vi "I(V)_MFLI_PK_v4.0_measureR_phase.vi"() -> ()   [LabVIEW 2016]
uses:
  Labview Drivers/MFLI/LabOneLabVIEW-22.02.26577/LabOneLabVIEW-22.02.26577/Zurich Instruments LabOne/Public/Data/ziTypeDemodSampleSingle.ctl
  Labview Drivers/MFLI/LabOneLabVIEW-22.02.26577/LabOneLabVIEW-22.02.26577/Zurich Instruments LabOne/Public/Configure/ziSetValueDouble.vi
  Labview Drivers/MFLI/LabOneLabVIEW-22.02.26577/LabOneLabVIEW-22.02.26577/Zurich Instruments LabOne/Public/Configure/ziGetValueDemodSampleEx.vi
  Labview Drivers/MFLI/LabOneLabVIEW-22.02.26577/LabOneLabVIEW-22.02.26577/Zurich Instruments LabOne/Zurich Instruments LabOne.lvlib
panel:
  out "Iphase (deg)":dbl=-16.59997463839791 format="%#_13g"
  out "Vphase (deg)":dbl=40.57455732074348 format="%#_13g"
  out "Set Voltage(V)":dbl=4.384062043356605 format="%#_13g"
  out "Time(s)":dbl=185.322 format="%#_13g"
  out "Demod Sample Out 2":T1={"Timestamps (ticks)"=217071890701310, "X (Vrms)"=5.764492493379272e-06, "Y (Vrms)"=-1.7187028687058897e-06, "Osc Phase (deg)"=1.9746167692057917, "Freq (Hz)"=7.919000069023241, "DIO"=0, "AuxIn0 (V)"=-0.0006693530012853444, "AuxIn1 (V)"=0.0, "Trigger"=256}
  out "Demod Sample Out":T1={"Timestamps (ticks)"=217071887690750, "X (Vrms)"=8.75456933556226e-07, "Y (Vrms)"=7.498226005787958e-07, "Osc Phase (deg)"=5.4774618983426535, "Freq (Hz)"=7.919000069023241, "DIO"=0, "AuxIn0 (V)"=-0.001673382503213361, "AuxIn1 (V)"=-0.0006673162570223212, "Trigger"=512}
  in  "MFLI Current source/Voltage reader":string="DEV4496"
  out "Imeas (A)":dbl=6.015256707500007e-06
  out "Vmeas (V)":dbl=1.1526746179431637e-06
  in  "Folder":path=path "D:/Heng/Nb3Br8_JJ/Sb.3_NBVJ01/20210115"
  in  "wait (ms) [Should be > TC]":u32=1000
  out "I vs V":cluster{dbl, "Field Reading":dbl}[](graph)=[{2.1337108522522826e-07, "Field Reading"=1.0007121497539348e-06}, {2.0018204953851064e-08, "Field Reading"=1.0969598663661376e-07}, {3.474074033482476e-08, "Field Reading"=1.9016075130631681e-07}, {5.6400419155691035e-08, "Field Reading"=2.706780203266455e-07}, {7.134741663483111e-08, "Field Reading"=3.625194153695155e-07}, {8.711957733763268e-08, "Field Reading"=4.6186456260881066e-07}, {1.039613386460647e-07, "Field Reading"=5.541771498802743e-07}, {1.290159481540569e-07, "Field Reading"=6.517488283090827e-07}, {1.442006622421336e-07, "Field Reading"=7.441421685111633e-07}, {1.6579779771841864e-07, "Field Reading"=8.4200282004452e-07}, {1.7667431320194624e-07, "Field Reading"=9.371894272094692e-07}, {2.0346799660082097e-07, "Field Reading"=1.0346819690568719e-06}, {2.1275449478314156e-07, "Field Reading"=1.1273455634288892e-06}, {2.2792303722372882e-07, "Field Reading"=1.2246113813938451e-06}, {2.506226161778463e-07, "Field Reading"=1.3169699353558023e-06}, {2.6686786096204173e-07, "Field Reading"=1.4106741902497636e-06}, {2.979630377408132e-07, "Field Reading"=1.5068897992871093e-06}, {3.1162936250255217e-07, "Field Reading"=1.6013785409354697e-06}, {3.2854904168138843e-07, "Field Reading"=1.7007967107121696e-06}, {3.4501678279448686e-07, "Field Reading"=1.7932741209540488e-06}, {3.5732655253185603e-07, "Field Reading"=1.891133061059139e-06}, {3.7678513716337806e-07, "Field Reading"=1.9837632139333797e-06}, {3.8857693765173823e-07, "Field Reading"=2.078638757139878e-06}, {4.070455630330932e-07, "Field Reading"=2.1777621608691614e-06}, {4.3651006057087547e-07, "Field Reading"=2.270487653250022e-06}, {4.535609885287045e-07, "Field Reading"=2.364817703267964e-06}, {4.800092323465329e-07, "Field Reading"=2.4630513126122318e-06}, {4.872172260420143e-07, "Field Reading"=2.560612214294704e-06}, {5.029105394973937e-07, "Field Reading"=2.653407522930296e-06}, {5.207137968885614e-07, "Field Reading"=2.7508846993110185e-06}, {5.449974912672081e-07, "Field Reading"=2.8437164663468094e-06}, {5.549097834910874e-07, "Field Reading"=2.941117576580943e-06}, {5.789147944756835e-07, "Field Reading"=3.0334756142859178e-06}, {5.940331669154695e-07, "Field Reading"=3.130923358288321e-06}, {6.192662248173834e-07, "Field Reading"=3.223457045619671e-06}, {6.338859460756282e-07, "Field Reading"=3.3210140787077685e-06}, {6.617730672082958e-07, "Field Reading"=3.4134337904467758e-06}, {6.708744764433933e-07, "Field Reading"=3.511218639909905e-06}, {6.876034184888421e-07, "Field Reading"=3.6064791588715936e-06}, {7.081705825683568e-07, "Field Reading"=3.704194984998823e-06}, {7.341349902267621e-07, "Field Reading"=3.796795088130521e-06}, {7.500412173627324e-07, "Field Reading"=3.894221622472711e-06}, {7.635282212201655e-07, "Field Reading"=3.986359362120525e-06}, {7.839559208505005e-07, "Field Reading"=4.084105589459172e-06}, {7.991337007295971e-07, "Field Reading"=4.176440151889332e-06}, {8.175550663233945e-07, "Field Reading"=4.274041338897146e-06}, {8.360511976155764e-07, "Field Reading"=4.366718612721536e-06}, {8.595654269642977e-07, "Field Reading"=4.46481586459238e-06}, {8.846044621269243e-07, "Field Reading"=4.559710869350914e-06}, {8.902214589762566e-07, "Field Reading"=4.6535858762473605e-06}, {9.13930972707384e-07, "Field Reading"=4.751211544539011e-06}, {9.218629476317926e-07, "Field Reading"=4.843674806906942e-06}, {9.389346568153207e-07, "Field Reading"=4.94148963023105e-06}, {9.661788530141893e-07, "Field Reading"=5.0340339305698605e-06}, {9.734275114489362e-07, "Field Reading"=5.134274890899915e-06}, {9.91273930192609e-07, "Field Reading"=5.227194198108034e-06}, {1.0062090937222443e-06, "Field Reading"=5.324543514118811e-06}, {1.0324830232331714e-06, "Field Reading"=5.417068558459935e-06}, {1.0500453704719826e-06, "Field Reading"=5.514414049876445e-06}, {1.0818020141498576e-06, "Field Reading"=5.606738838727315e-06}, {1.0919981214621985e-06, "Field Reading"=5.943499955969014e-06}, {1.1041062115858416e-06, "Field Reading"=5.802825671371831e-06}, {1.12928896400331e-06, "Field Reading"=5.8897635364887065e-06}, {1.1492595887607054e-06, "Field Reading"=5.986959246668246e-06}, {1.1525838773614565e-06, "Field Reading"=6.079112281920131e-06}, {1.1732006667255544e-06, "Field Reading"=6.176765549637453e-06}, {1.193444625294635e-06, "Field Reading"=6.2693583656248445e-06}, {1.2101538188023656e-06, "Field Reading"=6.369277338631168e-06}, {1.2318147585414787e-06, "Field Reading"=6.462177680852612e-06}, {1.2413491771177379e-06, "Field Reading"=6.554239754143973e-06}, {1.2731631837142253e-06, "Field Reading"=6.653541226069562e-06}, {1.2825564782833625e-06, "Field Reading"=6.7454110623267924e-06}, {1.2992348301055137e-06, "Field Reading"=6.843115368447837e-06}, {1.316693256967963e-06, "Field Reading"=6.935702965257668e-06}, {1.343852132299077e-06, "Field Reading"=7.033596304342718e-06}, {0.0003223256295561193, "Field Reading"=7.130369502789653e-06}, {0.0010682796466779994, "Field Reading"=7.237712618778445e-06}, {0.0011012721847992696, "Field Reading"=7.315133567183911e-06}, {0.0011336841810168491, "Field Reading"=7.4123545054478695e-06}, {0.0011614058556892847, "Field Reading"=7.504304430827025e-06}, {0.001182885890671154, "Field Reading"=7.602366955750201e-06}, {0.001200897535521615, "Field Reading"=7.69976061587441e-06}, {0.00121594401470624, "Field Reading"=7.792677109208386e-06}, {0.0012308027651267619, "Field Reading"=7.886128685028496e-06}, {0.0012456418637471253, "Field Reading"=7.983615236672288e-06}, {0.001257564969772003, "Field Reading"=8.075760842161778e-06}, {0.0012690336996615858, "Field Reading"=8.170723157183957e-06}, {0.0012814644345765262, "Field Reading"=8.268995175290895e-06}, {0.0012910253378675095, "Field Reading"=8.363131378141633e-06}, {0.001301444806581894, "Field Reading"=8.45644533427298e-06}, {0.0013106148752890106, "Field Reading"=8.551458283635111e-06}, {0.0013201336522581891, "Field Reading"=8.65161959339898e-06}, {0.0013282012490195363, "Field Reading"=8.74416723601607e-06}, {0.0013370451945670784, "Field Reading"=8.841765835802203e-06}, {0.001345475691336453, "Field Reading"=8.933978266213217e-06}, {0.0013541642420234728, "Field Reading"=9.031643266856203e-06}, {0.0013602243952778926, "Field Reading"=9.123705087732138e-06}, {0.0013678078924535615, "Field Reading"=9.221510724442928e-06}, {0.0013749931650039048, "Field Reading"=9.319154251910434e-06}, {0.0013817418853904447, "Field Reading"=9.409423170522308e-06}, {0.0013877620940512577, "Field Reading"=9.50720467327743e-06}, {0.0013893900209027232, "Field Reading"=9.522740574798281e-06}, {0.0013841293323999348, "Field Reading"=9.444358568387913e-06}, {0.0013770955503089543, "Field Reading"=9.34786117205707e-06}, {0.0013707463881856257, "Field Reading"=9.255459479065146e-06}, {0.0013638010752030354, "Field Reading"=9.157506360964617e-06}, {0.001356127430849226, "Field Reading"=9.065389480276688e-06}, {0.0013481807501391138, "Field Reading"=8.967105386552946e-06}, {0.0013407950243109453, "Field Reading"=8.872574329619889e-06}, {0.0013327879049762552, "Field Reading"=8.780745564878272e-06}, {0.0013239176518001648, "Field Reading"=8.686977265427215e-06}, {0.0013146578852826479, "Field Reading"=8.586299385882446e-06}, {0.0013048672888862206, "Field Reading"=8.493635331032656e-06}, {0.0012950842712132512, "Field Reading"=8.395823484571033e-06}, {0.0012855051336405129, "Field Reading"=8.303455420153361e-06}, {0.001274818349601112, "Field Reading"=8.209679742685101e-06}, {0.0012618971608759537, "Field Reading"=8.109946125115199e-06}, {0.0012494525821266837, "Field Reading"=8.017364894823338e-06}, {0.001235685913286103, "Field Reading"=7.919657723881713e-06}, {0.0012216877307261714, "Field Reading"=7.824897358413329e-06}, {0.0012037516065472435, "Field Reading"=7.727435253164315e-06}, {0.0011875344677767074, "Field Reading"=7.634970945479442e-06}, {0.0011690885694813937, "Field Reading"=7.537773175917453e-06}, {0.001143867923079635, "Field Reading"=7.445625913634191e-06}, {0.0011139726709101221, "Field Reading"=7.348337041113834e-06}, {0.0010813147907609588, "Field Reading"=7.255852572757193e-06}, {0.0008158901453383064, "Field Reading"=7.15654215348316e-06}, {0.00014586885402730632, "Field Reading"=7.065078532967033e-06}, {6.672313176192101e-06, "Field Reading"=6.97131792702715e-06}, {1.311378694927265e-06, "Field Reading"=6.8592321760864306e-06}, {1.318127585000335e-06, "Field Reading"=6.78165201436255e-06}, {1.2916070805813707e-06, "Field Reading"=6.684382236814962e-06}, {1.2637872492482735e-06, "Field Reading"=6.591615618281428e-06}, {1.2510857193087697e-06, "Field Reading"=6.49373019741343e-06}, {1.2409566576000475e-06, "Field Reading"=6.399307801408899e-06}, {1.215389141425889e-06, "Field Reading"=6.305912312991265e-06}, {1.1948309642776338e-06, "Field Reading"=6.211147873874382e-06}, {1.1729714746286896e-06, "Field Reading"=6.112674813622632e-06}, {1.1526746179431637e-06, "Field Reading"=6.015256707500007e-06}]
  out "data":dbl[](array[numeric])=[1.1526746179431637e-06, 6.015256707500007e-06, 3.1500000000000066, 184.117, 40.57455732074348, -16.59997463839791]
  in  "Step":dbl[](array[numeric])=[0.02, 0.02, 0.02] min=-3000.0 max=3000.0 format="%.1e"
  in  "To":dbl[](array[numeric])=[1.2, -1.2, 0.0] min=-3000.0 max=3000.0 format="%.1e"
  in  "From":dbl[](array[numeric])=[0.0, 1.2, -1.2] min=-3000.0 max=3000.0 format="%.1e"
  in  "file name":string="002_NBVJ01_IV(8mK)_I16_R34_ac(13.3337Hz)"
  out "File path":path=path "D:/Heng/Nb3Br8_JJ/Sb.3_NBVJ01/20210115/002_NBVJ01_IV(8mK)_I16_R34_ac(13.3337Hz).dat"
  # ".dat"
  # "Set MFLI Voltage output (V)"
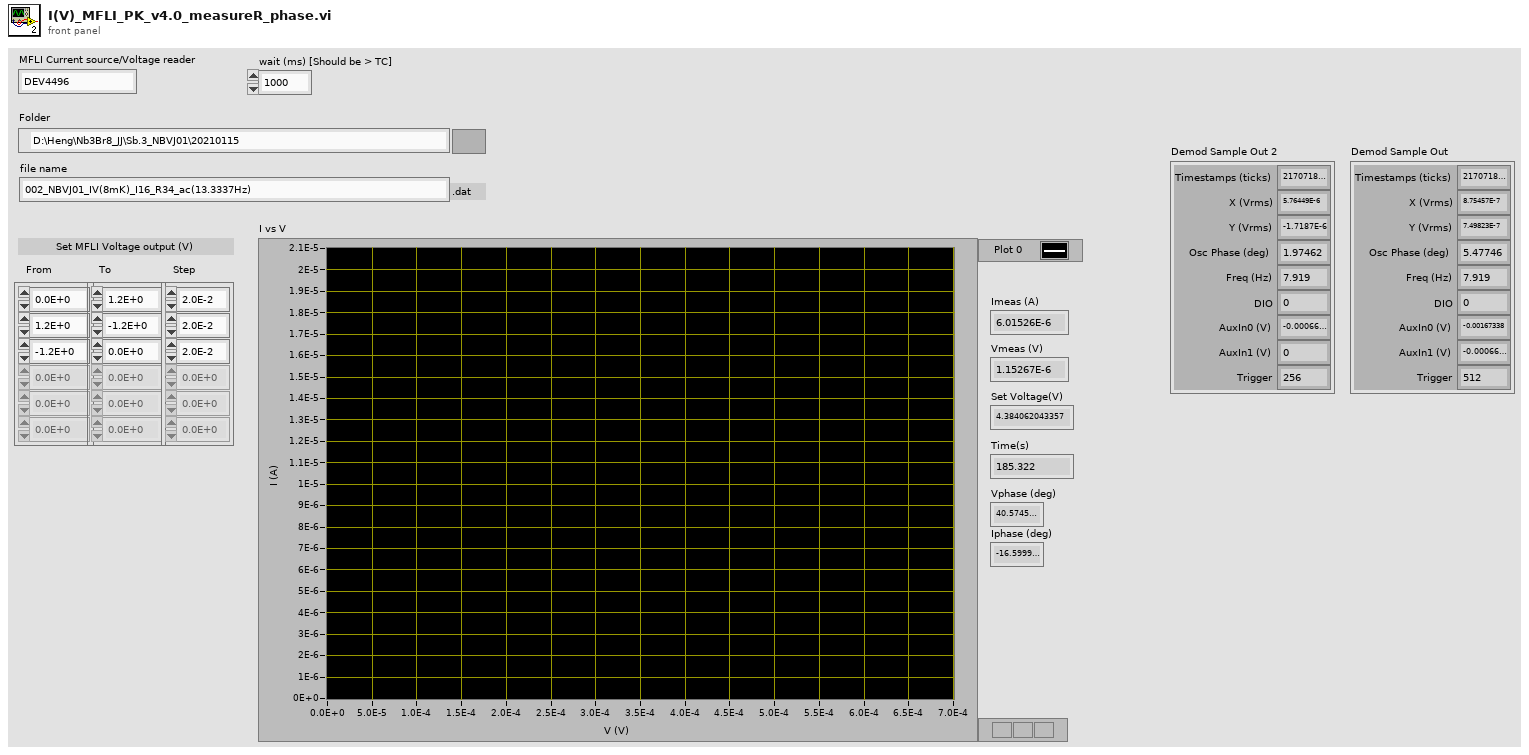
[diagram p1: front panel]
types:
  T1 = typedef "Zurich Instruments LabOne.lvlib/ziTypeDemodSampleSingle.ctl" = cluster{"Timestamps (ticks)":u64, "X (Vrms)":dbl, "Y (Vrms)":dbl, "Osc Phase (deg)":dbl, "Freq (Hz)":dbl, "DIO":u32, "AuxIn0 (V)":dbl, "AuxIn1 (V)":dbl, "Trigger":u32}
  T2 = enum16{"open", "replace", "create", "open or create", "replace or create", "replace or create with confirmation"}
  T3 = typedef "Zurich Instruments LabOne.lvlib/ziTypeHandle.ctl" = cluster{"handleValid":bool, "Conn":u64, "Path Prefix":string, "Handle":u64, "Connected":bool, "Clockbase(s)":dbl}
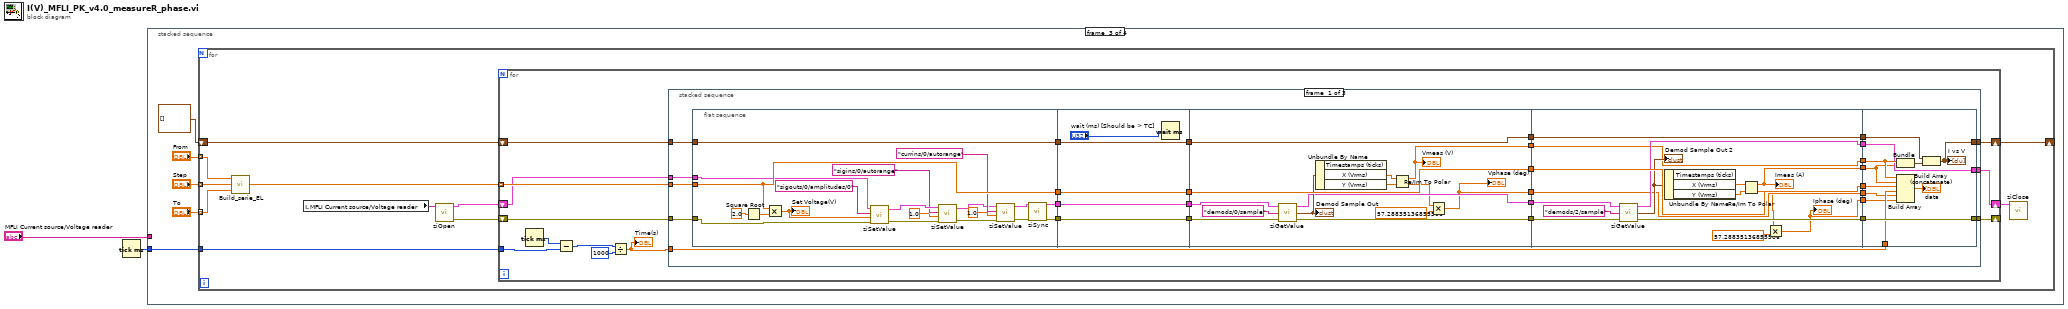
[diagram p0: block diagram]
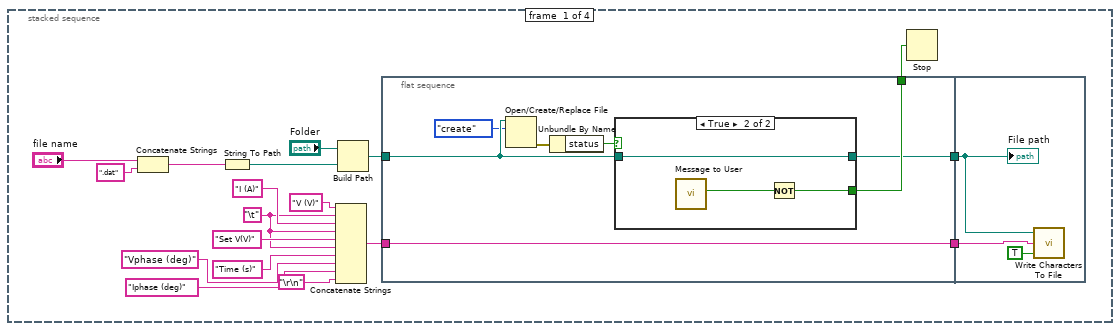
[diagram p2: hidden frame]
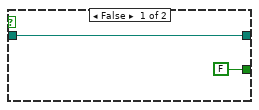
[diagram p3: hidden frame]
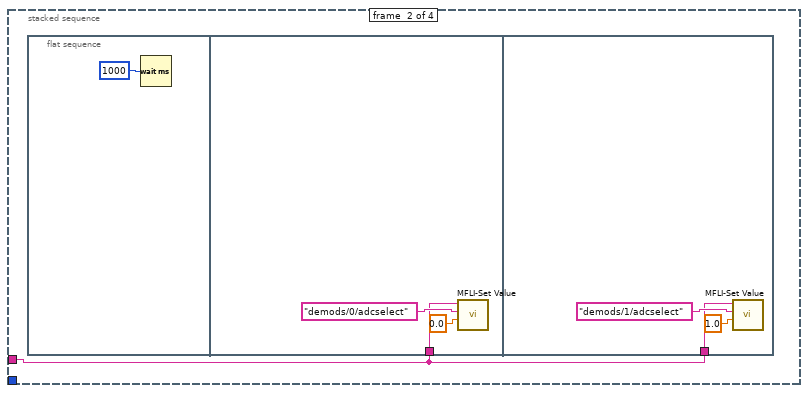
[diagram p4: hidden frame]
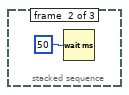
[diagram p5: hidden frame]
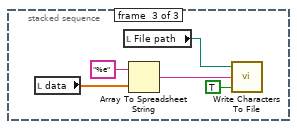
[diagram p6: hidden frame]
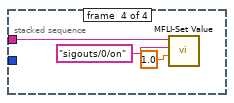
[diagram p7: hidden frame]
diagram:
  n1 = Tick Count (ms)() -> (millisecond timer value=w1:u32)
  n2 = stacked-sequence {
    tunnel: "MFLI Current source/Voltage reader" -> [_ w36 _ w175]
    tunnel: w1 -> [_ _ w44 _]
    frame #0 {
      w6 = "\t"
      n3 = Concatenate Strings("file name", ".dat" ("string")) -> (w17:string)
      n4 = String To Path(string=w17) -> (path=w9:path)
      n5 = Concatenate Strings("V (V)" ("string"), w6, "I (A)" ("string"), w6, "Set V(V)" ("string"), w6, "Time (s)", "Vphase (deg)", "Iphase (deg)", "\r\n") -> (w18:string)
      n6 = Build Path(base path="Folder", name or relative path=w9) -> (appended path=w8:path)
      n7 = flat-sequence {
        tunnel: w8 -> [w24]
        tunnel: w18 -> [w27]
        tunnel: [w27] -> w20
        tunnel: [w26] -> w15
        tunnel: [w25] -> w19
        tunnel: w20 -> [w34]
        tunnel: w19 -> [w33]
        frame #0 {
          n8 = Open/Create/Replace File(file path (use dialog)=w24, operation (0:open)=T2."create") -> (error out=w23:errorcluster)  [unwired: 4 in, 2 out]
          n9 = Unbundle By Name(w23) -> ("status"=w21:bool)
          n10 = case shown="True" w21 {
            tunnel: [FALSE ("Yes") w31] -> w26
            tunnel: [w28 w30] -> w25
            tunnel: w24 -> [w28 w30]
            frame False {
            }
            frame True {
              n11 = call "Message to User"() -> ("Yes"=w32:bool)  [unwired: 10 in, 1 out]
              n12 = Not(x=w32) -> (.not. x?=w31:bool)
            }
          }
        }
        frame #1 {
          n13 = call <vilib>:"Write Characters To File.vi"("append to file? (new file:F)"=TRUE, "character string"=w34, "file path (dialog if empty)"=w33) -> ()  [unwired: 2 in, 1 out]
          "File path" <- w33
        }
      }
      n14 = Stop(stop? (T)=w15) -> ()
    }
    frame #1 {
      n15 = flat-sequence {
        tunnel: w36 -> [w38]
        tunnel: w36 -> [w41]
        frame #0 {
          n16 = Wait (ms)(milliseconds to wait=u32 1000) -> ()  [unwired: 1 out]
        }
        frame #1 {
          n17 = call "MFLI-Set Value.vi"("Value"=0.0, "Path"="demods/0/adcselect", "MFLI Current source/Voltage reader"=w38) -> ()  [unwired: 9 in]
        }
        frame #2 {
          n18 = call "MFLI-Set Value.vi"("Value"=1.0, "Path"="demods/1/adcselect", "MFLI Current source/Voltage reader"=w41) -> ()  [unwired: 9 in]
        }
      }
    }
    frame #2 {
      n19 = for {
        tunnel: "From" -> [w56] mode=indexing
        tunnel: "To" -> [w55] mode=indexing
        tunnel: "Step" -> [w54] mode=indexing
        shift-right: [w58] -> _
        shift-left: cluster{dbl, "Field Reading":dbl}[] [] -> [w59]
        tunnel: w44 -> [w51]
        n20 = call "Build_serie_EL.vi"("end value"=w55, "increment"=w54, "start value"=w56) -> ("output array"=w57:dbl[])
        n21 = local read "MFLI Current source/Voltage reader"() -> (w53:string)
        n22 = call "ziOpen.vi"("Address"=w53) -> ("Error Out"=w49:errorcluster, "HandleOut"=w50:T3)  [unwired: 3 in, 1 out]
        n23 = for {
          tunnel: w57 -> [w71] mode=indexing
          shift-right: [w69] -> w58
          shift-left: w59 -> [w70]
          shift-right: [w66] -> w52
          shift-left: w50 -> [w68]
          shift-right: [w65] -> _
          shift-left: w49 -> [w67]
          tunnel: w51 -> [w61]
          n24 = Tick Count (ms)() -> (millisecond timer value=w62:u32)
          n25 = Subtract(x=w62, y=w61) -> (x-y=w63:u32)
          n26 = Divide(x=w63, y=1000) -> (x/y=w60:dbl)
          "Time(s)" <- w60
          n27 = stacked-sequence {
            tunnel: w71 -> [w99 _ _]
            tunnel: w70 -> [w100 _ _]
            tunnel: [w101 _ _] -> w69
            tunnel: w68 -> [w90 _ _]
            tunnel: w67 -> [w89 _ _]
            tunnel: [w79 _ _] -> w66
            tunnel: [w78 _ _] -> w65
            tunnel: w60 -> [w75 _ _]
            frame #0 {
              n28 = flat-sequence {
                tunnel: [w121] -> w96
                tunnel: [w120] -> w95
                tunnel: w99 -> [w120]
                tunnel: w100 -> [w121]
                tunnel: [w103] -> w92
                tunnel: [w104] -> w91
                tunnel: w90 -> [w106]
                tunnel: w89 -> [w105]
                tunnel: w96 -> [w126]
                tunnel: [w126] -> w98
                tunnel: w95 -> [w125]
                tunnel: [w125] -> w97
                tunnel: [w123] -> w94
                tunnel: [w122] -> w93
                tunnel: w92 -> [w122]
                tunnel: w91 -> [w123]
                tunnel: [w130] -> w88
                tunnel: [w140] -> w86
                tunnel: [w139] -> w84
                tunnel: w93 -> [w136]
                tunnel: w94 -> [w135]
                tunnel: w98 -> [w140]
                tunnel: w97 -> [w139]
                tunnel: [w134] -> w82
                tunnel: [w133] -> w81
                tunnel: [w127] -> w73
                tunnel: w88 -> [w148]
                tunnel: [w148] -> w87
                tunnel: w86 -> [w156]
                tunnel: [w156] -> w85
                tunnel: w84 -> [w155]
                tunnel: [w155] -> w83
                tunnel: w82 -> [w152]
                tunnel: w81 -> [w151]
                tunnel: [w150] -> w80
                tunnel: [w149] -> w77
                tunnel: [w145] -> w76
                tunnel: [w141] -> w74
                tunnel: w73 -> [w144]
                tunnel: [w144] -> w72
                tunnel: w87 -> [w167]
                tunnel: [w166] -> w101
                tunnel: w85 -> [w165]
                tunnel: w83 -> [w164]
                tunnel: [w163] -> w79
                tunnel: w80 -> [w163]
                tunnel: [w162] -> w78
                tunnel: w77 -> [w162]
                tunnel: w76 -> [w161]
                tunnel: w75 -> [w159]
                tunnel: w74 -> [w158]
                tunnel: w72 -> [w157]
                frame #0 {
                  n29 = Square Root(x=2.0) -> (sqrt(x)=w119:dbl)
                  n30 = Multiply(x=w120, y=w119) -> (x*y=w102:dbl)
                  "Set Voltage(V)" <- w102
                  n31 = call-poly "ziSetValue.vi"("Error In"=w105, "Value"=w102, "Path"="sigouts/0/amplitudes/0", "Handle In"=w106) -> ("Error Out"=w113:errorcluster, "Handle Out"=w116:T3)  [unwired: 1 in]
                  n32 = call-poly "ziSetValue.vi"("Error In"=w113, "Value"=1.0, "Path"="sigins/0/autorange", "Handle In"=w116) -> ("Error Out"=w109:errorcluster, "Handle Out"=w110:T3)  [unwired: 1 in]
                  n33 = call-poly "ziSetValue.vi"("Error In"=w109, "Value"=1.0, "Path"="currins/0/autorange", "Handle In"=w110) -> ("Error Out"=w107:errorcluster, "Handle Out"=w108:T3)  [unwired: 1 in]
                  n34 = call "ziSync.vi"("Handle In"=w108, "Error In"=w107) -> ("Handle Out"=w104:T3, "Error Out"=w103:errorcluster)  [unwired: 12 in]
                }
                frame #1 {
                  n35 = Wait (ms)(milliseconds to wait="wait (ms) [Should be > TC]") -> ()  [unwired: 1 out]
                }
                frame #2 {
                  n36 = call-poly "ziGetValue.vi"("error in"=w136, "Path"="demods/0/sample", "Handle In"=w135) -> ("error out"=w133:errorcluster, "Demod Sample Out"=w137:T1, "Handle Out"=w134:T3)
                  "Demod Sample Out" <- w137
                  n37 = Unbundle By Name(w137) -> ("X (Vrms)"=w132:dbl, "Y (Vrms)"=w131:dbl)  [unwired: 1 out]
                  n38 = Re/Im To Polar(2:w131, 3:w132) -> (0:w128:dbl, 1:w130:dbl)
                  "Vmeas (V)" <- w130
                  n39 = Multiply(x=w128, y=57.28835136855506) -> (x*y=w127:dbl)
                  "Vphase (deg)" <- w127
                }
                frame #3 {
                  n40 = call-poly "ziGetValue.vi"("error in"=w151, "Path"="demods/2/sample", "Handle In"=w152) -> ("error out"=w149:errorcluster, "Demod Sample Out"=w153:T1, "Handle Out"=w150:T3)
                  "Demod Sample Out 2" <- w153
                  n41 = Unbundle By Name(w153) -> ("X (Vrms)"=w146:dbl, "Y (Vrms)"=w147:dbl)  [unwired: 1 out]
                  n42 = Re/Im To Polar(2:w147, 3:w146) -> (0:w142:dbl, 1:w145:dbl)
                  "Imeas (A)" <- w145
                  n43 = Multiply(x=w142, y=57.28835136855506) -> (x*y=w141:dbl)
                  "Iphase (deg)" <- w141
                }
                frame #4 {
                  n44 = Bundle(w167, w161) -> (w160:cluster{dbl, dbl})  [unwired: 1 in]
                  n45 = Build Array(w167, w161, w164, w159, w157, w158) -> (→"data":dbl[])
                  n46 = Build Array (concatenate)(w165, w160) -> (w166:cluster{dbl, "Field Reading":dbl}[])
                  "I vs V" <- w166
                }
              }
            }
            frame #1 {
              n47 = Wait (ms)(milliseconds to wait=u32 50) -> ()  [unwired: 1 out]
            }
            frame #2 {
              n48 = local read "data"() -> (w170:dbl[])
              n49 = local read "File path"() -> (w172:path)
              n50 = Array To Spreadsheet String(array=w170, 3:"%e" ("format string")) -> (spreadsheet string=w173:string)  [unwired: 1 in]
              n51 = call <vilib>:"Write Characters To File.vi"("append to file? (new file:F)"=TRUE, "character string"=w173, "file path (dialog if empty)"=w172) -> ()  [unwired: 2 in, 1 out]
            }
          }
        }
        n52 = call "ziClose.vi"("Handle In"=w52) -> ()  [unwired: 1 in, 4 out]
      }
    }
    frame #3 {
      n53 = call "MFLI-Set Value.vi"("Value"=1.0, "Path"="sigouts/0/on", "MFLI Current source/Voltage reader"=w175) -> ()  [unwired: 9 in]
    }
  }
